vi "Read Visible_.vi"(8 "error in (no error)":errorcluster, 11 "Visible Assertion in":refnum<class "Visible Assertion.lvclass">) -> (0 "error out":errorcluster, 2 "Visible?":bool, 3 "Visible Assertion out":refnum<class "Visible Assertion.lvclass">)   [LabVIEW 2020, in "MacroAssert.lvlib" / "Visible Assertion.lvclass"]
uses:
  Visible Assertion.lvclass
  Visible Assertion.lvclass/Visible Assertion.ctl
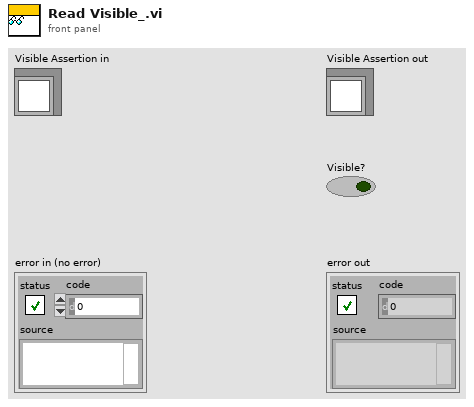
[diagram p1: front panel]
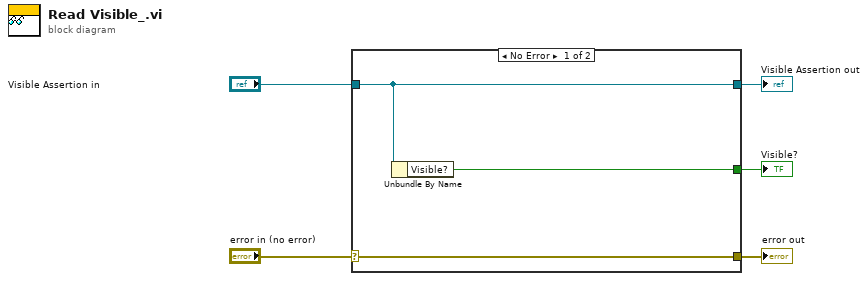
[diagram p0: block diagram]
diagram:
  n1 = case shown="No Error" "error in (no error)" {
    selector: "error in (no error)" -> [w8 w9]
    tunnel: [w8 w9] -> w4
    tunnel: [w7 w10] -> w2
    tunnel: "Visible Assertion in" -> [w7 w10]
    tunnel: [w6 _] -> w1
    frame No Error {
      n2 = Unbundle By Name(w7) -> ("Visible?"=w6:bool)
    }
    frame Error {
    }
  }
  "error out" <- w4
  "Visible Assertion out" <- w2
  "Visible?" <- w1
